vi "FTW-ProjectItemManager-AddToWriteTransaction.vi"(0 "Project Item Manager":refnum<class "FTW-ProjectItemManager.lvclass">, 5 "Tag":string, 7 "Value":variant, 11 "error in":errorcluster) -> (4 "Project Item Manager out":refnum<class "FTW-ProjectItemManager.lvclass">, 15 "error out":errorcluster)   [LabVIEW 2012, in "FTW-ProjectItemManager.lvclass"]
uses:
  FTW-ProjectItemManager.lvclass
  FTW-ProjectItemManager.lvclass/FTW-ProjectItemManager.ctl
panel:
  # "Inputs"
  # "Outputs"
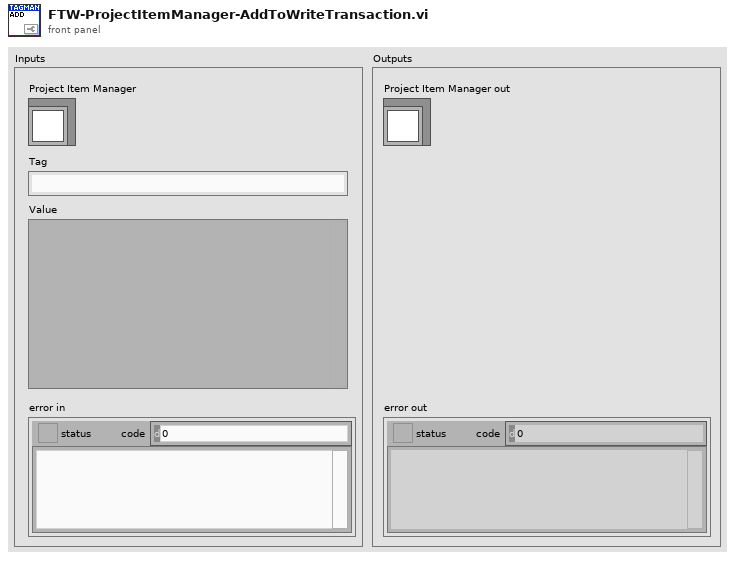
[diagram p1: front panel]
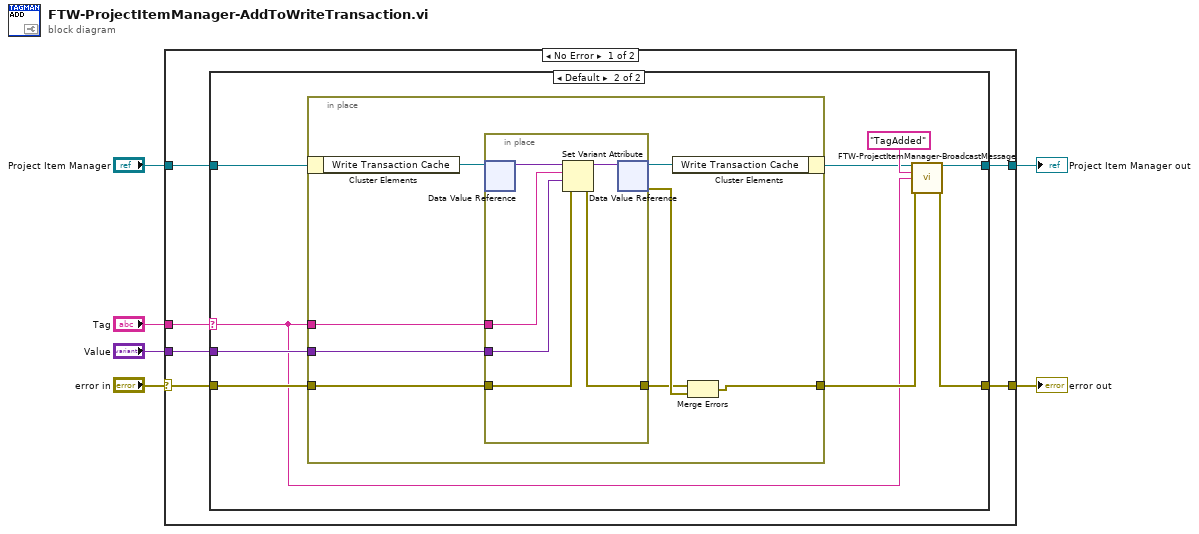
[diagram p0: block diagram]
diagram:
  n1 = case shown="No Error" "error in" {
    selector: "error in" -> [w12 w39]
    tunnel: [w11 w39] -> w6
    tunnel: [w8 w38] -> w4
    tunnel: "Project Item Manager" -> [w9 w38]
    tunnel: "Tag" -> [w7 _]
    tunnel: "Value" -> [w10 _]
    frame No Error {
      n2 = case shown="Default" w7 {
        selector: w7 -> [_ w15]
        tunnel: w12 -> [w13 w23]
        tunnel: [w13 w17] -> w11
        tunnel: w10 -> [_ w22]
        tunnel: w9 -> [w14 w21]
        tunnel: [w14 w18] -> w8
        frame "" {
        }
        frame Default {
          n3 = in-place {
            in-place-border: w23 -> [w31]
            in-place-border: [w24] -> w16
            in-place-border: w15 -> [w25]
            in-place-border: w22 -> [w30]
            n4 = in-place-cluster #1(w21) -> ("Write Transaction Cache"=w29:refnum<data-value>)
            n5 = in-place {
              in-place-border: w31 -> [w37]
              in-place-border: [w36] -> w26
              in-place-border: w25 -> [w35]
              in-place-border: w30 -> [w34]
              n6 = in-place-dvr #2(w29) -> (w33:variant)  [unwired: 1 out]
              n7 = Set Variant Attribute(Variant=w33, name=w35, value=w34, error in=w37) -> (Variant out=w32:variant, error out=w36:errorcluster)  [unwired: 1 out]
              n8 = in-place-dvr #2(w32) -> (w28:refnum<data-value>, w27:errorcluster)
            }
            n9 = in-place-cluster #1("Write Transaction Cache"=w28) -> (w19:refnum<class "FTW-ProjectItemManager.lvclass">)
            n10 = Merge Errors(w26, w27) -> (w24:errorcluster)
          }
          n11 = call "FTW-ProjectItemManager-BroadcastMessage.vi"("Project Item Manager"=w19, "Action Performed"="TagAdded", "Payload"=w15, "error in"=w16) -> ("Project Item Manager out"=w18:refnum<class "FTW-ProjectItemManager.lvclass">, "error out"=w17:errorcluster)  [unwired: 10 in]
        }
      }
    }
    frame Error {
    }
  }
  "error out" <- w6
  "Project Item Manager out" <- w4
